vi "Encode_Base_Info.vi"(8 "error in (no error)":errorcluster, 9 "Refresh Token":string, 10 "Authentication Info":T1, 11 "OAuth in":refnum<class "OAuth.lvclass">) -> (0 "error out":errorcluster, 3 "OAuth out":refnum<class "OAuth.lvclass">)   [LabVIEW 2016, in "OAuth.lvclass"]
uses:
  OAuth.lvclass
  OAuth.lvclass/OAuth.ctl
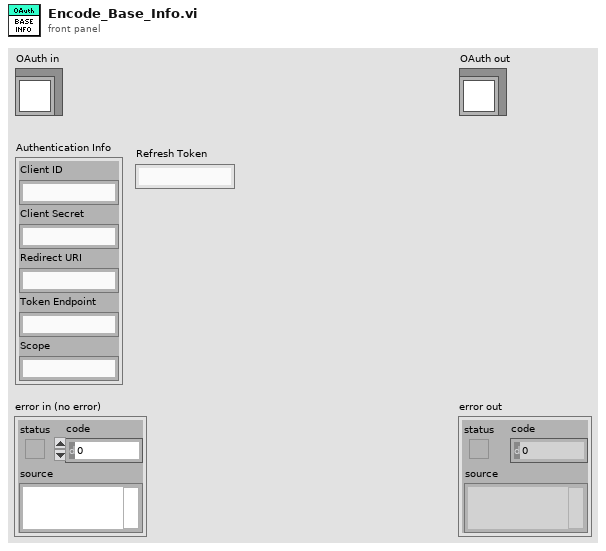
[diagram p1: front panel]
types:
  T1 = cluster{"Client ID":string, "Client Secret":string, "Redirect URI":string, "Token Endpoint":string, "Scope":string}
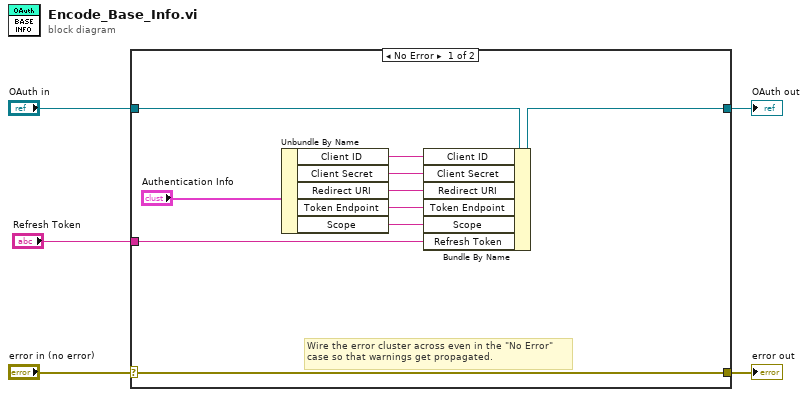
[diagram p0: block diagram]
diagram:
  n1 = case shown="No Error" "error in (no error)" {
    selector: "error in (no error)" -> [w15 w17]
    tunnel: [w15 w17] -> w4
    tunnel: [w13 w16] -> w2
    tunnel: "OAuth in" -> [w14 w16]
    tunnel: "Refresh Token" -> [w6 _]
    frame No Error {
      # "Wire the error cluster across even in the \"No Error\"\ncase so that warnings get propagated."
      n2 = Unbundle By Name("Authentication Info") -> ("Client ID"=w7:string, "Client Secret"=w8:string, "Redirect URI"=w9:string, "Token Endpoint"=w10:string, "Scope"=w11:string)
      n3 = Bundle By Name(cluster=w14, "Client ID"=w7, "Client Secret"=w8, "Redirect URI"=w9, "Token Endpoint"=w10, "Scope"=w11, "Refresh Token"=w6) -> (w13:refnum<class "OAuth.lvclass">)
    }
    frame Error {
    }
  }
  "error out" <- w4
  "OAuth out" <- w2
